vi "Get Custom Device Details.vi"(8 "error in":errorcluster, 11 "Device Reference in":u64 format="%.0x") -> (0 "error out":errorcluster, 3 "Data Reference out":u64=18446744073709551615 format="%.0x", 5 "Custom Device Details":T1)   [LabVIEW 2026, in "Template Engine.lvlib"]
uses:
  Template Engine.lvlib
  <vilib>/NI VeriStand/Custom Device API/Custom Device API.lvlib
  <vilib>/NI VeriStand/Custom Device API/Get Item Property (String).vi
  <vilib>/NI VeriStand/Custom Device API/Get Item Property (Variant).vi
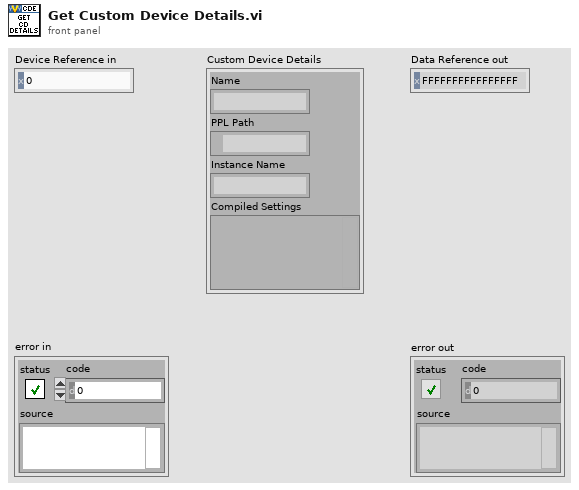
[diagram p1: front panel]
types:
  T1 = cluster{"Name":string, "PPL Path":path, "Instance Name":string, "Compiled Settings":variant}
  T2 = typedef "Custom Device API.lvlib/Custom Device Item Ref.ctl" = u64
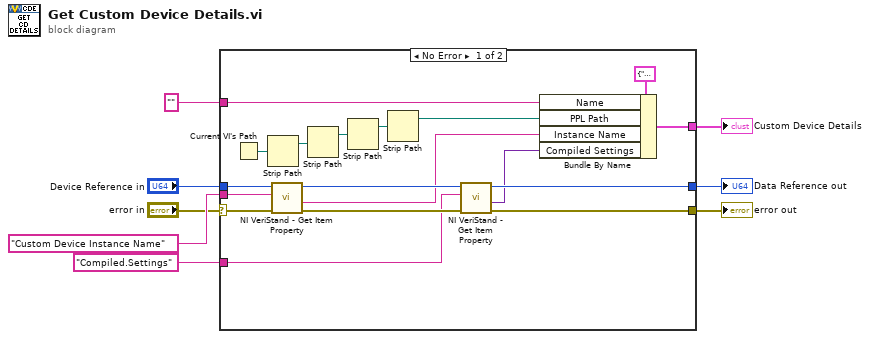
[diagram p0: block diagram]
diagram:
  n1 = case shown="No Error" "error in" {
    selector: "error in" -> [w21 w28]
    tunnel: "Device Reference in" -> [w26 w27]
    tunnel: "Custom Device Instance Name" ("Property Name") -> [w25 _]
    tunnel: "Compiled.Settings" ("Property Name") -> [w22 _]
    tunnel: [w16 w28] -> w1
    tunnel: [w15 w27] -> w2
    tunnel: "" ("CD.Name") -> [w11 _]
    tunnel: [w10 _] -> w3
    frame No Error {
      n2 = Current VI's Path() -> (path=w17:path)
      n3 = Strip Path(path=w17) -> (stripped path=w18:path)  [unwired: 1 out]
      n4 = call-poly <vilib>:"NI VeriStand - Get Item Property.vi"("error in (no error)"=w21, "Property Name"=w25, "Item Ref in"=w26) -> ("error out"=w24:errorcluster, "Value"=w13:string, "Item Ref out"=w23:T2)  [unwired: 5 in, 1 out]
      n5 = Strip Path(path=w18) -> (stripped path=w19:path)  [unwired: 1 out]
      n6 = Strip Path(path=w19) -> (stripped path=w20:path)  [unwired: 1 out]
      n7 = Strip Path(path=w20) -> (stripped path=w12:path)  [unwired: 1 out]
      n8 = call-poly <vilib>:"NI VeriStand - Get Item Property.vi"("error in (no error)"=w24, "Property Name"=w22, "Item Ref in"=w23) -> ("error out"=w16:errorcluster, "Value"=w14:variant, "Item Ref out"=w15:T2)  [unwired: 5 in, 1 out]
      n9 = Bundle By Name(cluster=T1 {"Name"="", "PPL Path"=path "", "Instance Name"="", "Compiled Settings"=variant} ("Cluster"), "Name"=w11, "PPL Path"=w12, "Instance Name"=w13, "Compiled Settings"=w14) -> (w10:T1)
    }
    frame Error {
    }
  }
  "Custom Device Details" <- w3
  "Data Reference out" <- w2
  "error out" <- w1
